vi "CalculatePowerPursuit.vi"(6 "Reset":bool, 9 "Gains":T1={"FFV"=0.0, "Vel PID"={"P"=1.0, "I"=0.01, "D"=0.0}} {"Vel PID"."D" format="%.3f"; "Vel PID"."I" format="%.3f"; "Vel PID"."P" format="%.3f"}, 10 "Vel":dbl, 11 "Target Vel":dbl) -> (3 "Power":dbl)   [LabVIEW 2016]
uses:
  <vilib>/addons/control/pid/pid.llb/PID (DBL).vi
  <vilib>/addons/control/pid/NI_PID_pid.lvlib
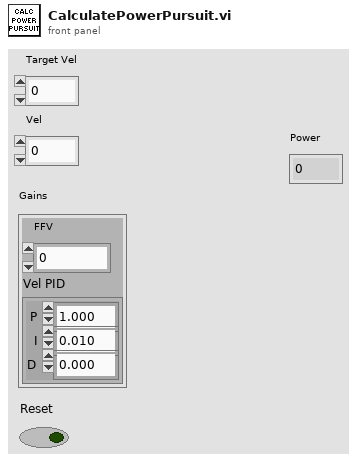
[diagram p1: front panel]
types:
  T1 = cluster{"FFV":dbl, "Vel PID":cluster{"P":dbl, "I":dbl, "D":dbl}}
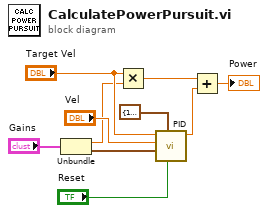
[diagram p0: block diagram]
diagram:
  n1 = Unbundle("Gains") -> ("FFV"=w5:dbl, "Vel PID"=w7:cluster{"P":dbl, "I":dbl, "D":dbl})
  n2 = Multiply(x="Target Vel", y=w5) -> (x*y=w3:dbl)
  n3 = call-poly <vilib>:"PID.vi"("reinitialize? (F)"="Reset", "output range"=cluster{"output high":dbl, "output low":dbl} {"output high"=1.0, "output low"=-1.0}, "PID gains"=w7, "process variable"="Vel", "setpoint"="Target Vel") -> ("output"=w2:dbl)  [unwired: 5 in, 1 out]
  n4 = Add(x=w3, y=w2) -> (x+y=→"Power":dbl)
